vi "Minutos_a_horas.vi"(11 "Duracion":i32) -> (3 "String":string)   [LabVIEW 2017]
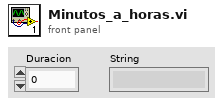
[diagram p1: front panel]
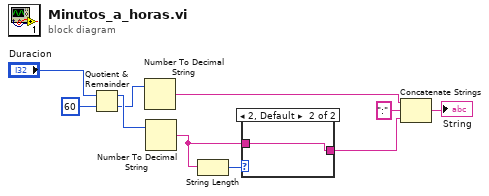
[diagram p0: block diagram]
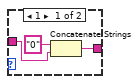
[diagram p2: hidden frame]
diagram:
  n1 = Quotient & Remainder(x="Duracion", y=60) -> (x-y*floor(x/y)=w9:i32, floor(x/y)=w8:i32)
  n2 = Number To Decimal String(number=w8) -> (decimal integer string=w5:string)  [unwired: 1 in]
  n3 = Number To Decimal String(number=w9) -> (decimal integer string=w2:string)  [unwired: 1 in]
  n4 = String Length(string=w2) -> (length=w3:i32)
  n5 = case shown="2, Default" w3 {
    tunnel: w2 -> [w12 w14]
    tunnel: [w11 w14] -> w1
    frame 1 {
      n6 = Concatenate Strings("0" ("string"), w12) -> (w11:string)
    }
    frame 2, Default {
    }
  }
  n7 = Concatenate Strings(w5, ":" ("string"), w1) -> (→"String":string)
